vi "Colour.vi"(9 "result":string, 11 "colourRef":refnum<vi>) -> (3 "colourRef 2":refnum<vi>)   [LabVIEW 2020]
uses:
  Global_Variable/Global.vi
panel:
  out "错误输出":errorcluster
  in  "result 2":string
  in  "黄灯":bool
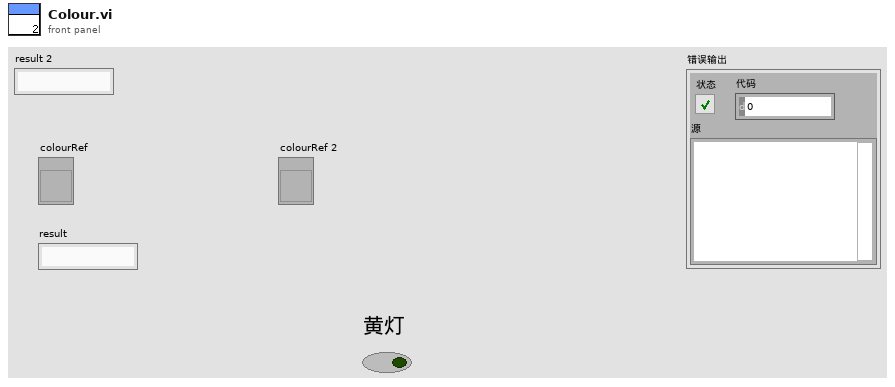
[diagram p1: front panel]
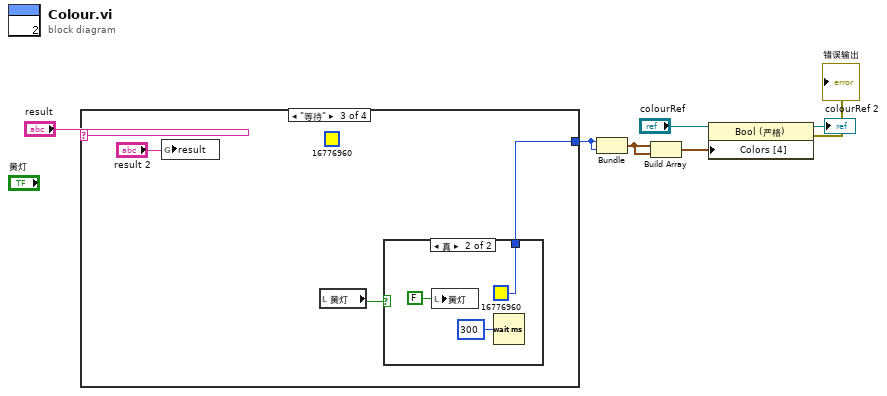
[diagram p0: block diagram]
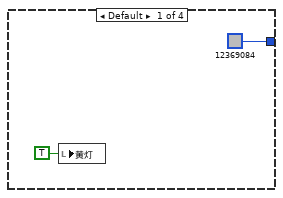
[diagram p2: hidden frame]
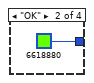
[diagram p3: hidden frame]
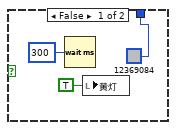
[diagram p4: hidden frame]
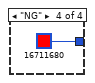
[diagram p5: hidden frame]
diagram:
  n1 = case shown="\"等待\"" "result" {
    tunnel: [u32 12369084 u32 6618880 w11 u32 16711680] -> w7
    frame Default {
      n2 = local write "黄灯"(TRUE ("黄灯")) -> ()
    }
    frame "OK" {
    }
    frame "等待" {
      (unwired) u32 16776960
      n3 = global write "Global.vi" "result"("result 2") -> ()
      n4 = local read "黄灯"() -> (w13:bool)
      n5 = case shown="真" w13 {
        tunnel: [u32 12369084 u32 16776960] -> w11
        frame False {
          n6 = Wait (ms)(milliseconds to wait=u32 300 ("等待时间（毫秒）")) -> ()  [unwired: 1 out]
          n7 = local write "黄灯"(TRUE ("黄灯")) -> ()
        }
        frame True {
          n8 = local write "黄灯"(FALSE ("黄灯")) -> ()
          n9 = Wait (ms)(milliseconds to wait=u32 300 ("等待时间（毫秒）")) -> ()  [unwired: 1 out]
        }
      }
    }
    frame "NG" {
    }
  }
  n10 = Bundle(w7, w7) -> (w6:cluster{u32, u32})  [unwired: 1 in]
  n11 = Build Array(w6, w6) -> (w2:cluster{u32, u32}[])
  n12 = property class="Bool (严格)"(reference="colourRef", "Colors [4]"=w2) -> (reference out=→"colourRef 2":refnum<vi>, error out=→"错误输出":errorcluster)  [unwired: 1 in]
